vi "Test Namer with Folder default folder with extension no label.vi"   [LabVIEW 2020, in "Namer.Tests.lvclass"]
uses:
  Namer.Tests.lvclass
  Source/Approval Tests/Namer with Folder/Namer with Folder.lvclass
  Source/Approval Tests/Naming Data/Naming Data.lvclass
  Source/Approval Tests/Naming Data/Naming Data.lvclass/Naming Data.ctl
  Source/Approval Tests/Naming Data/Write Test VI Name.vi
  Source/Approval Tests/Naming Data/Write Extension.vi
  <vilib>/addons/_JKI Toolkits/Caraya/classes/Assert/Assert Equal Value and Type_Variant.vi
  <vilib>/addons/_JKI Toolkits/Caraya/classes/Test/Test.lvclass
  <vilib>/addons/_JKI Toolkits/Caraya/classes/Assert/Assert.lvclass
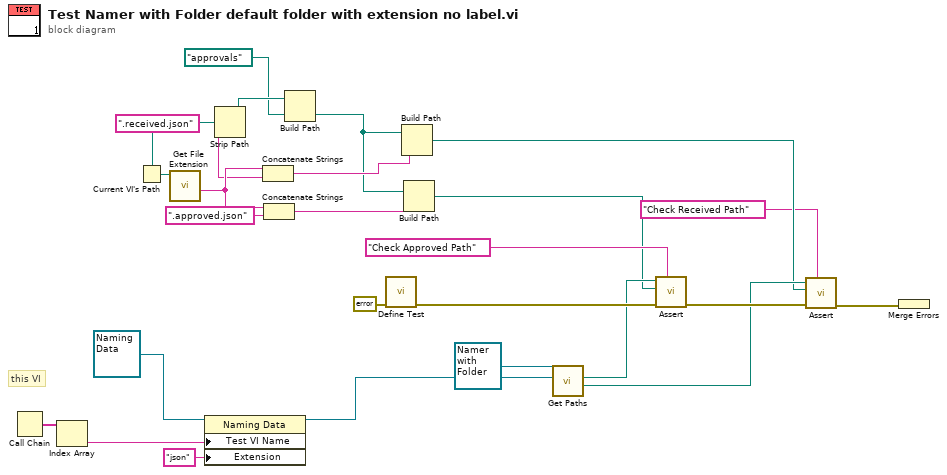
[diagram p0: block diagram]
diagram:
  # "this VI"
  n1 = Call Chain() -> (call chain=w20:string[])
  n2 = Index Array(array=w20) -> (element=w19:string)  [unwired: 1 in]
  n3 = Current VI's Path() -> (path=w13:path)
  n4 = call <vilib>:"Get File Extension.vi"("file"=w13) -> ("filename without extension"=w12:string)  [unwired: 6 in, 4 out]
  n5 = property on="Property Node" class="Naming Data"(reference=refnum<class "Naming Data.lvclass"> refnum ("Naming Data"), "Test VI Name"=w19, "Extension"="json") -> (reference out=w18:refnum<class "Naming Data.lvclass">)  [unwired: 1 in, 1 out]
  n6 = Strip Path(path=w13) -> (stripped path=w2:path)  [unwired: 1 out]
  n7 = Concatenate Strings(w12, ".received.json" ("string")) -> (w9:string)
  n8 = Concatenate Strings(w12, ".approved.json" ("string")) -> (w8:string)
  n9 = Build Path(base path=w2, name or relative path=path "approvals") -> (appended path=w3:path)
  n10 = call <vilib>:"Define Test.vi"("error in (no error)"=errorcluster {"status"=FALSE, "code"=0, "source"=""}) -> ("error out"=w24:errorcluster)  [unwired: 9 in, 1 out]
  n11 = Build Path(base path=w3, name or relative path=w9) -> (appended path=w7:path)
  n12 = Build Path(base path=w3, name or relative path=w8) -> (appended path=w6:path)
  n13 = call-dynamic "Get Paths.vi"("Naming Data"=w18, "Namer with Folder in"=refnum<class "Namer with Folder.lvclass"> refnum ("Approval Tests:Namer with SubFolder.lvclass")) -> ("Received Path"=w14:path, "Approved Path"=w15:path)  [unwired: 6 in, 2 out]
  n14 = call-poly <vilib>:"Assert.vi"("Label"="Check Approved Path" ("Label (VI Title)"), "error in (no error)"=w24, "Y"=w6, "X"=w15) -> ("error out"=w17:errorcluster)  [unwired: 6 in, 1 out]
  n15 = call-poly <vilib>:"Assert.vi"("Label"="Check Received Path" ("Label (VI Title)"), "error in (no error)"=w17, "Y"=w7, "X"=w14) -> ("error out"=w16:errorcluster)  [unwired: 6 in, 1 out]
  n16 = Merge Errors(w16) -> ()  [unwired: 1 out]
